vi "例程1-Random generate.vi"() -> ()   [LabVIEW 2013]
panel:
  out "数字(0-1)":dbl
  out "循环次数":i32
  in  "停止":bool
  out "波形图表":dbl(graph)
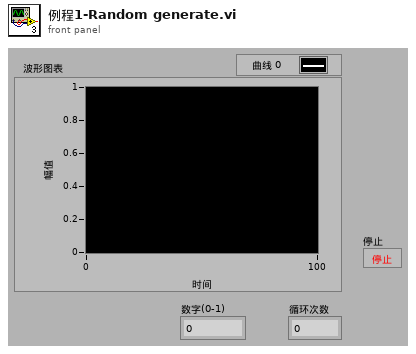
[diagram p1: front panel]
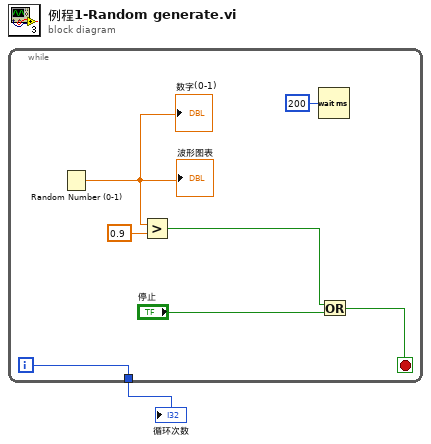
[diagram p0: block diagram]
diagram:
  n1 = while {
    tunnel: [w2] -> w1
    i -> [w2]
    stop <- w3 stop-if-true
    n2 = Random Number (0-1)() -> (number: 0 to 1=w6:dbl)
    "波形图表" <- w6
    "数字(0-1)" <- w6
    n3 = Greater?(x=w6, y=0.9) -> (0:w5:bool)
    n4 = Wait (ms)(milliseconds to wait=u32 200 ("等待时间（毫秒）")) -> ()  [unwired: 1 out]
    n5 = Or(x=w5, y="停止") -> (x .or. y?=w3:bool)
  }
  "循环次数" <- w1
